vi "Calculate Mean.vi"(5 "Waveform":waveform(dbl)) -> (2 "Waveform Mean":waveform(dbl))   [LabVIEW 2013, in "Empirical Mode Decomposition.lvlib"]
uses:
  Empirical Mode Decomposition.lvlib
  <vilib>/gmath/NI_Gmath.lvlib
panel:
  out "Signal":waveform(dbl)(graph)
  out "Minima":waveform(dbl)(graph)
  out "Maxima":waveform(dbl)(graph)
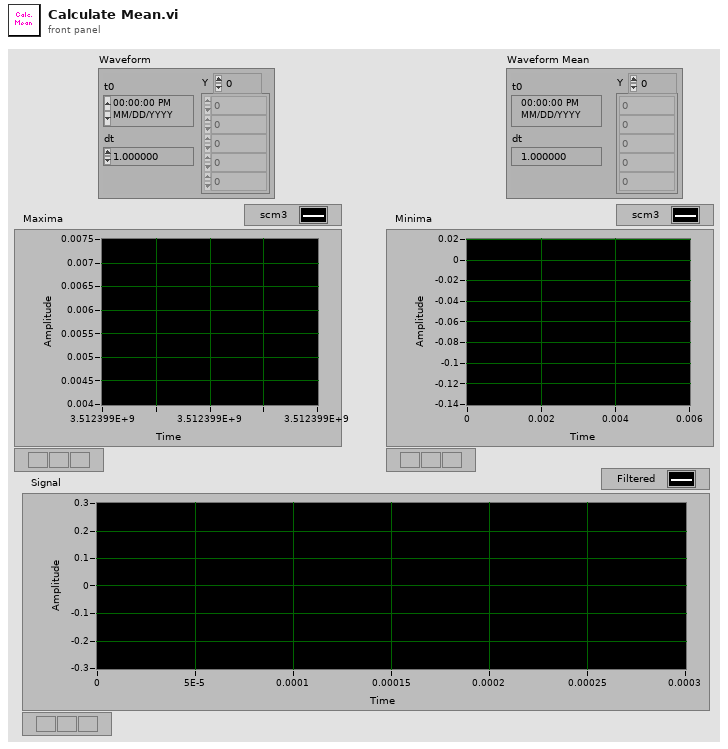
[diagram p1: front panel]
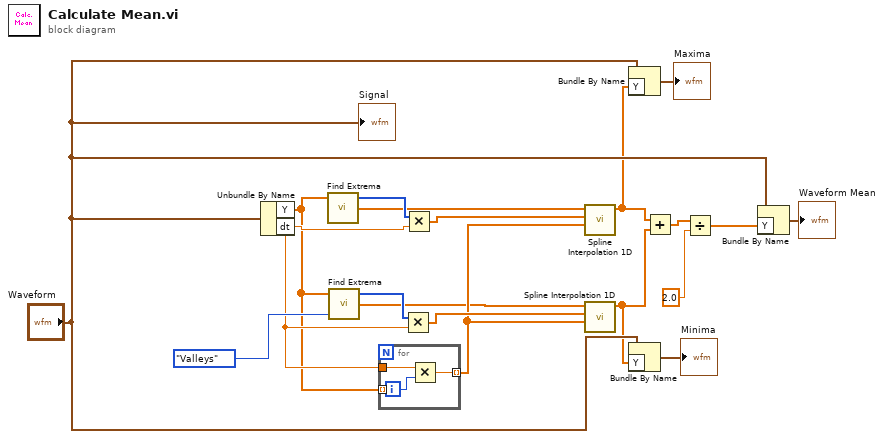
[diagram p0: block diagram]
diagram:
  n1 = Unbundle By Name("Waveform") -> ("Y"=w4:dbl[], "dt"=w8:dbl)
  n2 = call "Find Extrema.vi"("Array"=w4) -> ("Amplitudes"=w2:dbl[], "Indicies"=w12:u32[])  [unwired: 2 in, 1 out]
  n3 = call "Find Extrema.vi"("peaks/valleys"=enum32{"Peaks", "Valleys"}."Valleys", "Array"=w4) -> ("Amplitudes"=w1:dbl[], "Indicies"=w11:u32[])  [unwired: 1 in, 1 out]
  n4 = for {
    tunnel: w8 -> [w22]
    tunnel: [w20] -> w3 mode=indexing
    tunnel: w4 -> [_] mode=indexing
    i -> [w21]
    n5 = Multiply(x=w22, y=w21) -> (x*y=w20:dbl)
  }
  n6 = Multiply(x=w11, y=w8) -> (x*y=w5:dbl[])
  n7 = Multiply(x=w12, y=w8) -> (x*y=w6:dbl[])
  n8 = call <vilib>:"Spline Interpolation 1D.vi"("xi"=w3, "X"=w6, "Y"=w2) -> ("yi"=w13:dbl[])  [unwired: 6 in, 2 out]
  n9 = call <vilib>:"Spline Interpolation 1D.vi"("xi"=w3, "X"=w5, "Y"=w1) -> ("yi"=w9:dbl[])  [unwired: 6 in, 2 out]
  n10 = Bundle By Name(cluster="Waveform", "Y"=w13) -> (→"Maxima":waveform(dbl))
  n11 = Bundle By Name(cluster="Waveform", "Y"=w9) -> (→"Minima":waveform(dbl))
  n12 = Add(x=w13, y=w9) -> (x+y=w19:dbl[])
  n13 = Divide(x=w19, y=2.0) -> (x/y=w17:dbl[])
  n14 = Bundle By Name(cluster="Waveform", "Y"=w17) -> (→"Waveform Mean":waveform(dbl))
  "Signal" <- "Waveform"
